vi "Wait (wrapper).vi"(7 "milliseconds to wait (200)":u32=200, 8 "error in (no error)":errorcluster) -> (0 "error out":errorcluster)   [LabVIEW 2015]
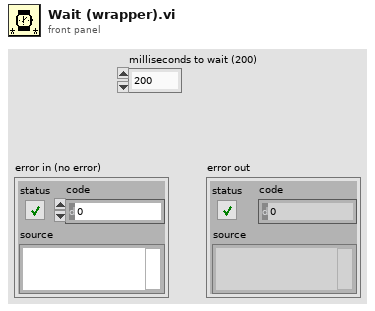
[diagram p1: front panel]
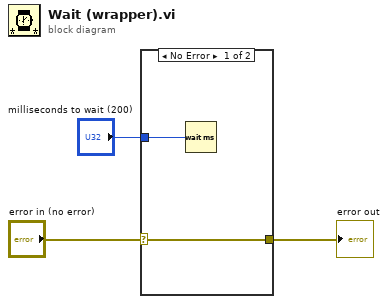
[diagram p0: block diagram]
diagram:
  n1 = case shown="No Error" "error in (no error)" {
    selector: "error in (no error)" -> [w4 w6]
    tunnel: "milliseconds to wait (200)" -> [w5 _]
    tunnel: [w4 w6] -> w1
    frame No Error {
      n2 = Wait (ms)(milliseconds to wait=w5) -> ()  [unwired: 1 out]
    }
    frame Error {
    }
  }
  "error out" <- w1
